vi "Agilent DMM Set Stimulus.vi"(7 "Agilent DMM":T2, 8 "error in (no error)":errorcluster, 10 "Stimulus":T1, 11 "VISA Resource Name":refnum<visa-resource-name>) -> (0 "error out":errorcluster {"code" format="%.0x"}, 3 "dup VISA Resource Name":refnum<visa-resource-name>)   [LabVIEW 2011]
uses:
  TypeDefs/Agilent DMM Instrument Info.ctl
  tests/DC Attenuation/TypeDefs/DCA Stimulus Parameters.ctl
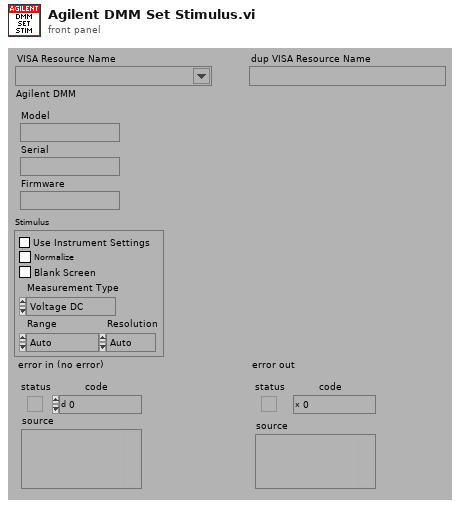
[diagram p1: front panel]
types:
  T1 = typedef "DCA Stimulus Parameters.ctl" = cluster{"Use Instrument":bool, "Normalize":bool, "Blank Screen":bool, "Measurement Type":enum16{"Voltage DC", "Voltage DC Ratio", "Voltage AC", "Current DC", "Current AC", "Resistance", "Fresistance", "Frequency", "Period", "Continuity", "Diode"}, "Range":enum16{"Auto", "Minimum", "Maximum", "100", "1,000", "10,000", "100,000", "1,000,000", "10,000,000", "100,000,000"}, "Resolution":enum16{"Auto", "4 1/2", "5 1/2", "6 1/2"}}
  T2 = typedef "Agilent DMM Instrument Info.ctl" = cluster{"Model":string, "Serial":string, "Firmware":string}
  T3 = enum16{"Auto", "Minimum", "Maximum", "100", "1,000", "10,000", "100,000", "1,000,000", "10,000,000", "100,000,000"}
  T4 = enum16{"Voltage DC", "Voltage DC Ratio", "Voltage AC", "Current DC", "Current AC", "Resistance", "Fresistance", "Frequency", "Period", "Continuity", "Diode"}
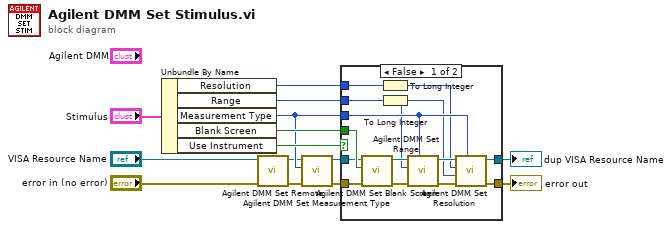
[diagram p0: block diagram]
diagram:
  n1 = Unbundle By Name("Stimulus") -> ("Resolution"=w10:enum16{"Auto", "4 1/2", "5 1/2", "6 1/2"}, "Range"=w9:T3, "Measurement Type"=w7:T4, "Blank Screen"=w13:bool, "Use Instrument"=w8:bool)
  n2 = call "Agilent DMM Set Remote.vi"("error in (no error)"="error in (no error)", "VISA Resource Name"="VISA Resource Name") -> ("error out"=w4:errorcluster, "dup VISA Resource Name"=w3:refnum<visa-resource-name>)  [unwired: 8 out]
  n3 = call "Agilent DMM Set Measurement Type.vi"("error in (no error)"=w4, "Measurement Type"=w7, "VISA Resource Name"=w3) -> ("error out"=w6:errorcluster, "dup VISA Resource Name"=w5:refnum<visa-resource-name>)  [unwired: 7 out]
  n4 = case shown="False" w8 {
    tunnel: w13 -> [w28 _]
    tunnel: w5 -> [w20 w30]
    tunnel: w6 -> [w19 w29]
    tunnel: [w26 w30] -> w12
    tunnel: [w25 w29] -> w11
    tunnel: w10 -> [w23 _]
    tunnel: w7 -> [w22 _]
    tunnel: w9 -> [w21 _]
    frame False {
      n5 = call "Agilent DMM Set Blank Screen.vi"("error in (no error)"=w19, "Blank Screen"=w28, "VISA Resource Name"=w20) -> ("error out"=w17:errorcluster, "dup VISA Resource Name"=w18:refnum<visa-resource-name>)  [unwired: 7 out]
      n6 = To Long Integer(number=w23) -> (32bit integer=w15:i32)
      n7 = To Long Integer(number=w21) -> (32bit integer=w16:i32)
      n8 = call "Agilent DMM Set Range.vi"("Measurement Type"=w22, "error in (no error)"=w17, "Range"=w16, "VISA Resource Name"=w18) -> ("error out"=w24:errorcluster, "dup VISA Resource Name"=w27:refnum<visa-resource-name>)  [unwired: 1 in, 5 out]
      n9 = call "Agilent DMM Set Resolution.vi"("Measurement Type"=w22, "error in (no error)"=w24, "Range"=w16, "Resolution"=w15, "VISA Resource Name"=w27) -> ("error out"=w25:errorcluster, "dup VISA Resource Name"=w26:refnum<visa-resource-name>)  [unwired: 5 out]
    }
    frame True {
    }
  }
  "error out" <- w11
  "dup VISA Resource Name" <- w12
